vi "UpdateVoltResultFixture.vi"(7 "Auto FR/FL":bool=TRUE, 8 "Test Name":string(combo)="Door Lock", 9 "Result 2":bool=TRUE, 10 "Result 1":bool=TRUE, 11 "Fixture Array Input":u16[](array[numeric])) -> (0 "Result":bool, 3 "Fixture Array Output":u16[](array[numeric]))   [LabVIEW 2017]
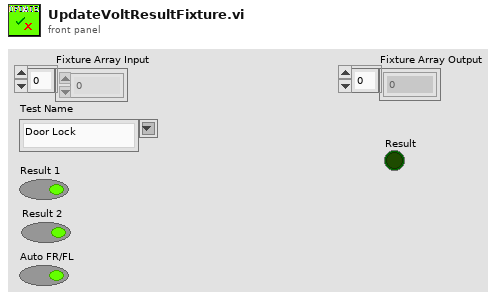
[diagram p1: front panel]
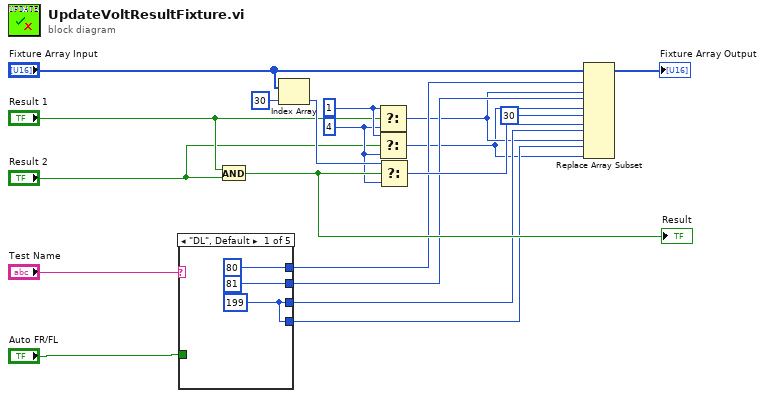
[diagram p0: block diagram]
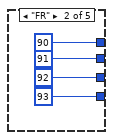
[diagram p2: hidden frame]
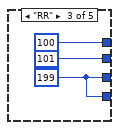
[diagram p3: hidden frame]
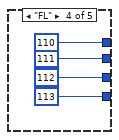
[diagram p4: hidden frame]
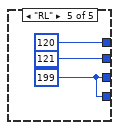
[diagram p5: hidden frame]
diagram:
  w15 = 4
  w19 = 1
  n1 = case shown="\"DL\", Default" "Test Name" {
    tunnel: [80 ("index") 90 ("index") 100 ("index") 110 ("index") 120 ("index")] -> w9
    tunnel: [81 ("index") 91 ("index") 101 ("index") 111 ("index") 121 ("index")] -> w8
    tunnel: "Auto FR/FL" -> [_ _ _ _ _]
    tunnel: [w20 92 ("index") w27 112 ("index") w34] -> w4
    tunnel: [w20 93 ("index") w27 113 ("index") w34] -> w3
    frame "DL", Default {
      w20 = 199 ("index")
    }
    frame "FR" {
    }
    frame "RR" {
      w27 = 199 ("index")
    }
    frame "FL" {
    }
    frame "RL" {
      w34 = 199 ("index")
    }
  }
  n2 = And(x="Result 1", y="Result 2") -> (x .and. y?=w17:bool)
  "Result" <- w17
  n3 = Index Array(array="Fixture Array Input", index=30) -> (element=w16:u16)
  n4 = Select(t=w19, s="Result 1", f=w15) -> (s? t:f=w2:i32)
  n5 = Select(t=w19, s="Result 2", f=w15) -> (s? t:f=w1:i32)
  n6 = Select(t=w16, s=w17, f=w15) -> (s? t:f=w13:i32)
  n7 = Replace Array Subset(array="Fixture Array Input", new element #1=w2, index #1=w9, new element #2=w1, index #2=w8, new element #3=w13, index #3=30 ("index"), new element #4=w2, index #4=w4, new element #5=w1, index #5=w3) -> (→"Fixture Array Output":u16[])
